vi "Initialize AO.vi"(8 "error in (no error)":errorcluster, 9 "AO Channel Setting":T1={"AO Channel name"=[], "output terminal configuration"=-1, "minimum value"=-10.0, "maximum value"=10.0, "units"=10348, "name to assign"=[]} {"units" items=["Volts"=10348, "From Custom Scale"=10065]; "maximum value" format="%0.2f"; "minimum value" format="%0.2f"; "output terminal configuration" items=["Default"=-1, "RSE"=10083, "Differential"=10106, "Pseudodifferential"=12529]}, 10 "DAQ Type":enum16{"Hardware", "Simulation"}(ring), 11 "Abstract in":refnum<class "Abstract.lvclass">) -> (0 "error out":errorcluster, 3 "Abstract out":refnum<class "Abstract.lvclass">)   [LabVIEW 2021, in "DAQ Hardware.lvlib" / "Abstract.lvclass"]
uses:
  Abstract.lvclass
  AO Channel Setting.ctl
  DAQ Hardware.lvlib
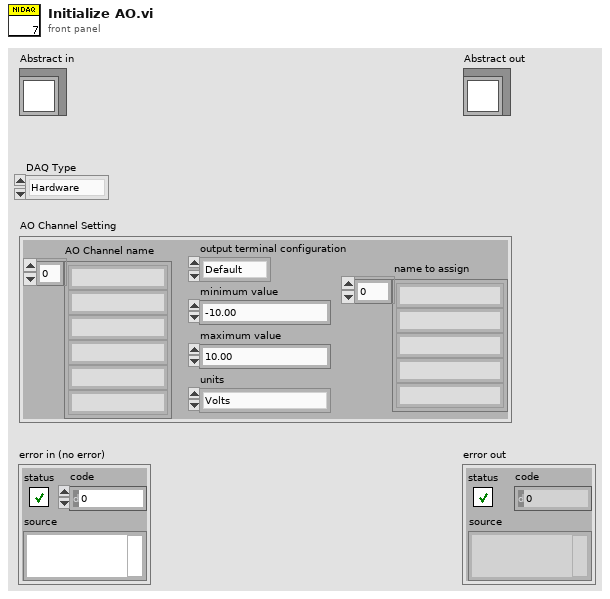
[diagram p1: front panel]
types:
  T1 = typedef "DAQ Hardware.lvlib/AO Channel Setting.ctl" = cluster{"AO Channel name":string[], "output terminal configuration":i32, "minimum value":dbl, "maximum value":dbl, "units":i32, "name to assign":string[]}
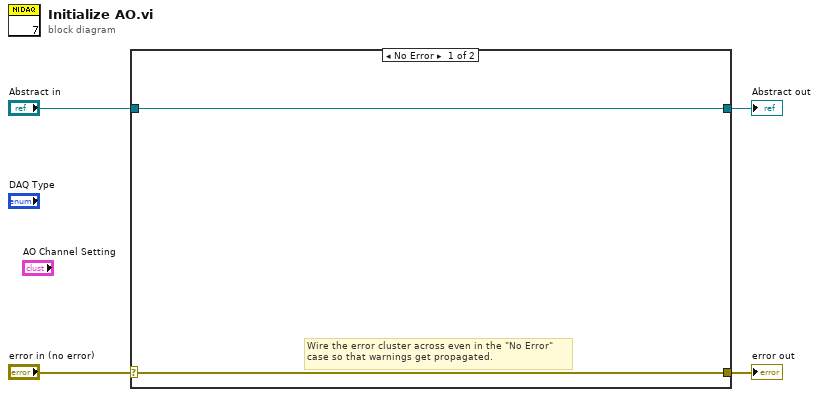
[diagram p0: block diagram]
diagram:
  n1 = case shown="No Error" "error in (no error)" {
    selector: "error in (no error)" -> [w5 w8]
    tunnel: [w5 w8] -> w3
    tunnel: [w6 w7] -> w1
    tunnel: "Abstract in" -> [w6 w7]
    frame No Error {
      # "Wire the error cluster across even in the \"No Error\"\ncase so that warnings get propagated."
    }
    frame Error {
    }
  }
  "error out" <- w3
  "Abstract out" <- w1
